vi "Joystick Notifier Set.vi"   [LabVIEW 2013]
uses:
  <vilib>/Rock Robotics/WPI/Joystick/WPI_JoystickGetSetRefNum.vi
types:
  T1 = typedef "WPI_JoystickDevRef.ctl" = cluster{"Device":T2}
  T2 = typedef "WPI_JoystickDeviceEnum.ctl" = enum16{"USB 1", "USB 2", "USB 3", "USB 4", "Kinect 1", "Kinect 2"}
  T3 = cluster{"axis 1 (x)":dbl, "axis 2 (y)":dbl, "axis 3 (throttle)":dbl, "axis 4":dbl, "axis 5":dbl, "axis 6":dbl}
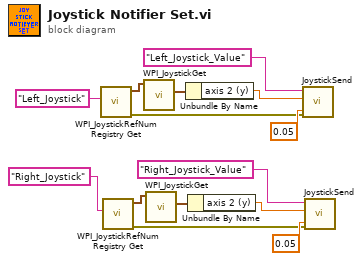
[diagram p0: block diagram]
diagram:
  n1 = call <vilib>:"WPI_JoystickRefNum Registry Get.vi"("refnum name"="Left_Joystick") -> ("error out"=w3:errorcluster, "JoystickDevRef"=w2:T1)  [unwired: 9 in]
  n2 = call <vilib>:"WPI_JoystickRefNum Registry Get.vi"("refnum name"="Right_Joystick") -> ("error out"=w10:errorcluster, "JoystickDevRef"=w9:T1)  [unwired: 9 in]
  n3 = call <vilib>:"WPI_JoystickGet.vi"("JoystickDevRef"=w2) -> ("Axes"=w4:T3)  [unwired: 4 in, 2 out]
  n4 = call <vilib>:"WPI_JoystickGet.vi"("JoystickDevRef"=w9) -> ("Axes"=w11:T3)  [unwired: 4 in, 2 out]
  n5 = Unbundle By Name(w4) -> ("axis 2 (y)"=w5:dbl)
  n6 = Unbundle By Name(w11) -> ("axis 2 (y)"=w12:dbl)
  n7 = call "JoystickSend.vi"("Epsilon"=0.05, "error in (no error)"=w3, "Joystick Value"=w5, "Notifier Name"="Left_Joystick_Value") -> ()  [unwired: 7 in, 1 out]
  n8 = call "JoystickSend.vi"("Epsilon"=0.05, "error in (no error)"=w10, "Joystick Value"=w12, "Notifier Name"="Right_Joystick_Value") -> ()  [unwired: 7 in, 1 out]
